vi "Motor Brake Control.vi"(8 "error in (no error)":errorcluster, 10 "Brake":bool, 11 "DAQ Ref Cluster in":T1) -> (0 "error out":errorcluster, 3 "DAQ Ref Cluster out":T1)   [LabVIEW 2021]
uses:
  Controls/DAQ Refnums.ctl
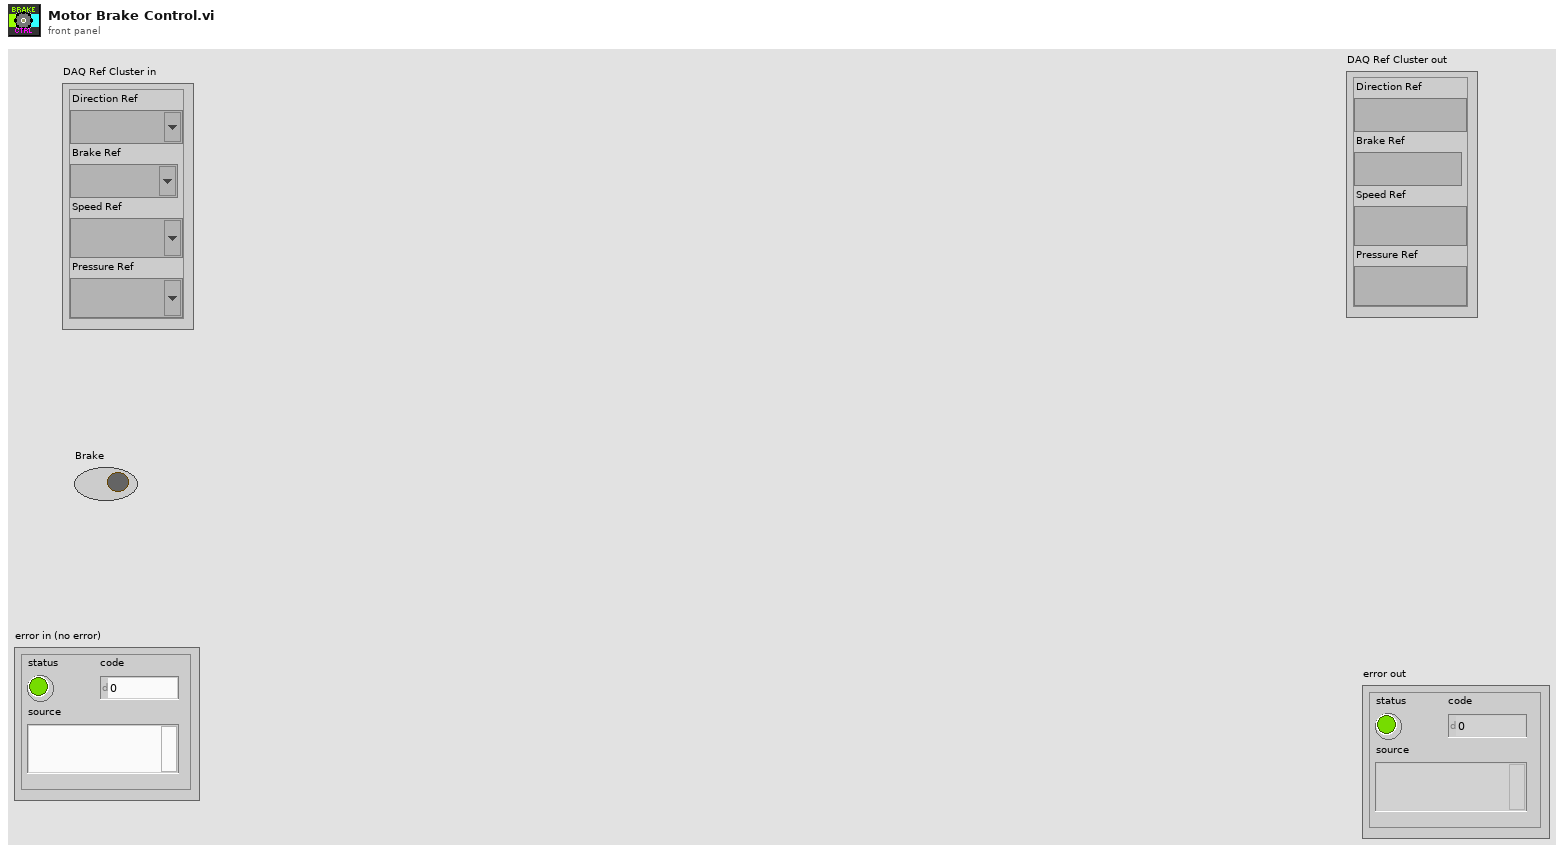
[diagram p1: front panel]
types:
  T1 = typedef "DAQ Refnums.ctl" = cluster{"Direction Ref":refnum<k21>, "Brake Ref":refnum<k21>, "Speed Ref":refnum<k21>, "Pressure Ref":refnum<k21>}
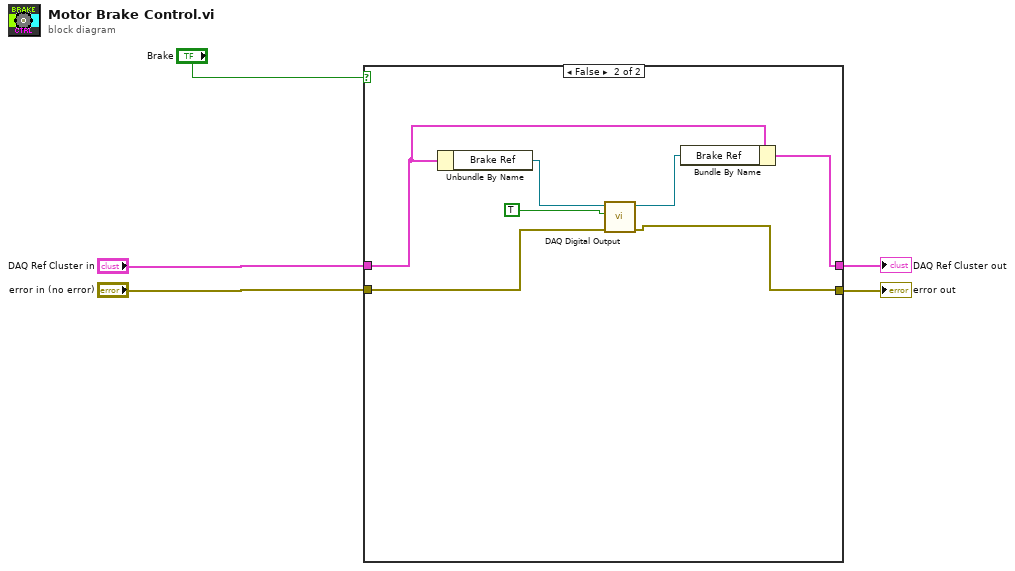
[diagram p0: block diagram]
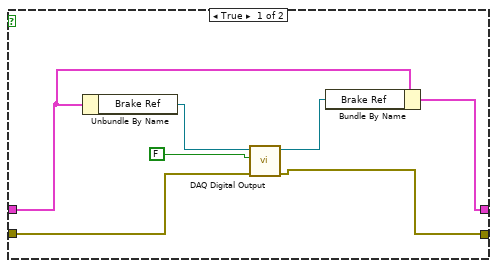
[diagram p2: hidden frame]
diagram:
  n1 = case shown="False" "Brake" {
    tunnel: "DAQ Ref Cluster in" -> [w8 w15]
    tunnel: "error in (no error)" -> [w7 w14]
    tunnel: [w9 w16] -> w4
    tunnel: [w6 w13] -> w5
    frame True {
      n2 = Unbundle By Name(w8) -> ("Brake Ref"=w11:refnum<k21>)
      n3 = call "DAQ Digital Output.vi"("error in"=w7, "data"=FALSE, "task/channels in"=w11) -> ("error out"=w6:errorcluster, "task out"=w10:refnum<k21>)  [unwired: 6 in, 1 out]
      n4 = Bundle By Name(cluster=w8, "Brake Ref"=w10) -> (w9:T1)
    }
    frame False {
      n5 = Unbundle By Name(w15) -> ("Brake Ref"=w18:refnum<k21>)
      n6 = call "DAQ Digital Output.vi"("error in"=w14, "data"=TRUE, "task/channels in"=w18) -> ("error out"=w13:errorcluster, "task out"=w17:refnum<k21>)  [unwired: 6 in, 1 out]
      n7 = Bundle By Name(cluster=w15, "Brake Ref"=w17) -> (w16:T1)
    }
  }
  "error out" <- w5
  "DAQ Ref Cluster out" <- w4
